vi "Read.vi"(6 "prioritize Cache? (F)":bool, 7 "Qualified Name":string, 8 "error in (no error)":errorcluster, 9 "Default Values":variant[](array[variant]), 10 "keys in":string[](array[string]), 11 "ConfigManager in":refnum<class "ConfigManager.lvclass">) -> (0 "error out":errorcluster, 1 "Values":variant[](array[variant]), 2 "keys":string[](array[string]), 3 "ConfigManager out":refnum<class "ConfigManager.lvclass">)   [LabVIEW 2013, in "CfgManager.lvlib" / "ConfigManager.lvclass"]
uses:
  ConfigManager.lvclass
  ConfigManager.lvclass/ConfigManager.ctl
  Encoding/Encoding.lvclass
  Encryption/Encryption.lvclass
  Serializer/Serializer.lvclass
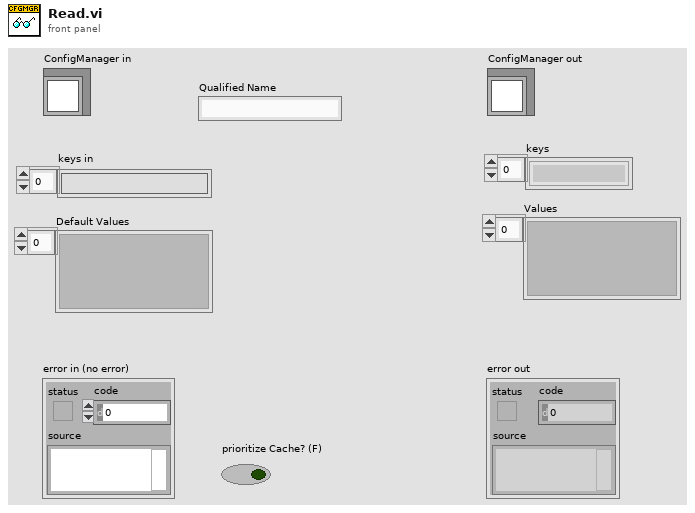
[diagram p1: front panel]
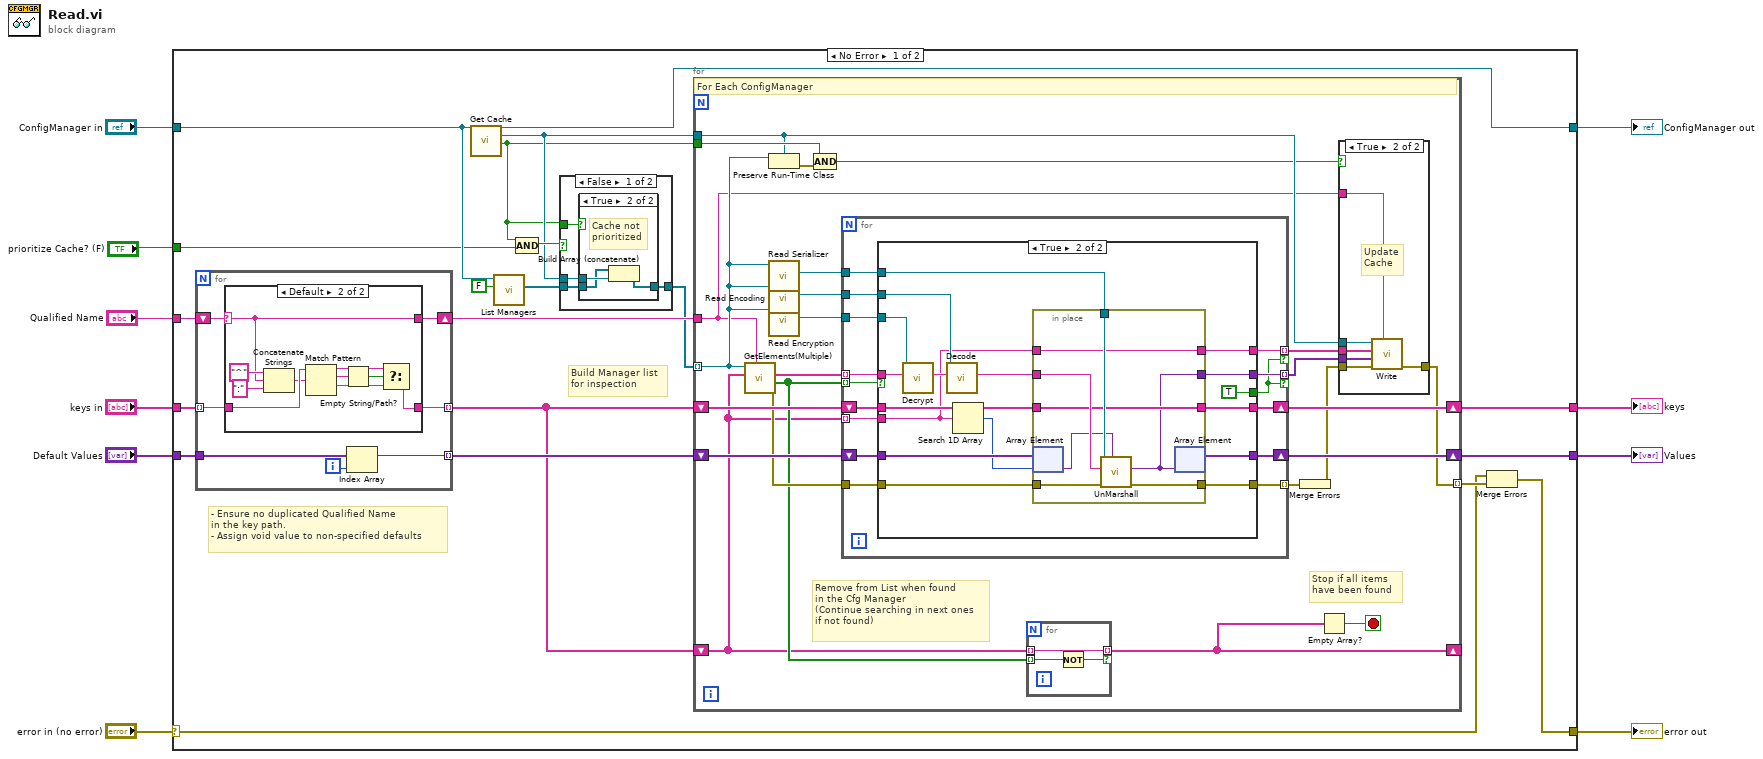
[diagram p0: block diagram]
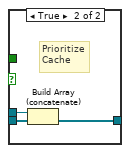
[diagram p3: hidden frame]
diagram:
  n1 = case shown="No Error" "error in (no error)" {
    selector: "error in (no error)" -> [w25 w141]
    tunnel: [w24 w141] -> w9
    tunnel: [w11 w140] -> w7
    tunnel: "ConfigManager in" -> [w18 w140]
    tunnel: "keys in" -> [w23 w138]
    tunnel: "Default Values" -> [w29 w139]
    tunnel: [w28 w139] -> w4
    tunnel: [w27 w138] -> w3
    tunnel: "Qualified Name" -> [w21 _]
    tunnel: "prioritize Cache? (F)" -> [w14 _]
    frame No Error {
      # "Build Manager list\nfor inspection"
      # "- Ensure no duplicated Qualified Name\nin the key path.\n- Assign void value to non-specified defaults"
      n2 = for {
        tunnel: w29 -> [w47]
        tunnel: [w46] -> w30 mode=indexing
        tunnel: w23 -> [w45] mode=indexing
        tunnel: [w42] -> w22 mode=indexing
        shift-right: [w43] -> w20
        shift-left: w21 -> [w44]
        i -> [w48]
        n3 = case shown="Default" w44 {
          selector: w44 -> [w50 w57]
          tunnel: w45 -> [w49 w60]
          tunnel: [w50 w57] -> w43
          tunnel: [w49 w51] -> w42
          frame "" {
          }
          frame Default {
            n4 = Concatenate Strings("^" ("string"), w57, ":" ("string")) -> (w59:string)
            n5 = Match Pattern(string=w60, regular expression=w59) -> (before substring=w54:string, match substring=w56:string, after substring=w53:string)  [unwired: 1 in, 1 out]
            n6 = Empty String/Path?(string/path=w56) -> (empty?=w55:bool)
            n7 = Select(t=w54, s=w55, f=w53) -> (s? t:f=w51:string)
          }
        }
        n8 = Index Array(array=w47, index=w48) -> (element=w46:variant)
      }
      n9 = call-dynamic "Get Cache.vi"("ConfigManager in"=w18) -> ("found?"=w12:bool, "Cache"=w13:refnum<class "ConfigManager.Cache.lvclass">, "ConfigManager out"=w11:refnum<class "ConfigManager.lvclass">)  [unwired: 8 in]
      n10 = call-dynamic "List Managers.vi"("Include Cache? (F)"=FALSE, "ConfigManager in"=w18) -> ("List"=w17:refnum<class "ConfigManager.lvclass">[])  [unwired: 8 in, 1 out]
      n11 = Compound Arithmetic op=AND(w12, w14) -> (w15:bool)
      n12 = case shown="False" w15 {
        tunnel: w13 -> [w33 w41]
        tunnel: w17 -> [w32 w40]
        tunnel: [w31 w39] -> w16
        tunnel: w12 -> [w34 _]
        frame False {
          n13 = case shown="True" w34 {
            tunnel: w33 -> [_ w38]
            tunnel: w32 -> [w35 w37]
            tunnel: [w35 w36] -> w31
            frame False {
              # "No cache\nfound"
            }
            frame True {
              # "Cache not\nprioritized"
              n14 = Build Array (concatenate)(w37, w38) -> (w36:refnum<class "ConfigManager.lvclass">[])
            }
          }
        }
        frame True {
          # "Prioritize\nCache"
          n15 = Build Array (concatenate)(w41, w40) -> (w39:refnum<class "ConfigManager.lvclass">[])
        }
      }
      n16 = for {
        tunnel: w16 -> [w75] mode=indexing
        shift-right: [w61] -> _
        shift-left: w22 -> [w63]
        shift-right: [w80] -> w28
        shift-left: w30 -> [w83]
        shift-right: [w81] -> w27
        shift-left: w22 -> [w82]
        tunnel: [w69] -> w26 mode=indexing
        tunnel: w20 -> [w67]
        tunnel: w13 -> [w72]
        tunnel: w12 -> [w73]
        stop <- w62 stop-if-true
        # "Remove from List when found\nin the Cfg Manager\n(Continue searching in next ones\nif not found)"
        # "Stop if all items\nhave been found"
        # "For Each ConfigManager"
        n17 = call-dynamic "GetElements(Multiple).vi"("Qualified Name"=w67, "keys"=w63, "ConfigManager in"=w75) -> ("error out"=w65:errorcluster, "Found"=w64:bool[], "Values"=w84:string[])  [unwired: 5 in, 1 out]
        n18 = Preserve Run-Time Class(object in=w75, 2:w72) -> (error out=w74:errorcluster)  [unwired: 1 in, 1 out]
        n19 = call "Read Serializer.vi"("ConfigManager in"=w75) -> ("Serializer"=w78:refnum<class "Serializer.lvclass">)  [unwired: 9 in, 1 out]
        n20 = call "Read Encoding.vi"("ConfigManager in"=w75) -> ("Encoding"=w79:refnum<class "Encoding.lvclass">)  [unwired: 9 in, 1 out]
        n21 = call "Read Encryption.vi"("ConfigManager in"=w75) -> ("Encryption"=w76:refnum<class "Encryption.lvclass">)  [unwired: 9 in, 1 out]
        n22 = Compound Arithmetic op=AND(w73, w74) -> (w66:bool)
        n23 = for {
          tunnel: w84 -> [w109] mode=indexing
          tunnel: w78 -> [w108]
          tunnel: w79 -> [w107]
          tunnel: w64 -> [w106] mode=indexing
          shift-right: [w103] -> w81
          shift-left: w82 -> [w105]
          shift-right: [w102] -> w80
          shift-left: w83 -> [w104]
          tunnel: w65 -> [w101]
          tunnel: [w100] -> w77 mode=indexing
          tunnel: w63 -> [w99] mode=indexing
          tunnel: w76 -> [w98]
          tunnel: [w97] -> w70 mode=indexing if=w95
          tunnel: [w96] -> w71 mode=indexing if=w95
          n24 = case shown="True" w106 {
            tunnel: w109 -> [_ w119]
            tunnel: w108 -> [_ w125]
            tunnel: w107 -> [_ w129]
            tunnel: w105 -> [w112 w122]
            tunnel: w104 -> [w111 w128]
            tunnel: [w112 w123] -> w103
            tunnel: [w111 w127] -> w102
            tunnel: w101 -> [w110 w121]
            tunnel: [w110 w120] -> w100
            tunnel: w99 -> [_ w114]
            tunnel: w98 -> [_ w117]
            tunnel: [_ w116] -> w97
            tunnel: [_ w115] -> w96
            tunnel: [_ TRUE] -> w95
            frame False {
            }
            frame True {
              n25 = call-dynamic "Decrypt.vi"("Encrypted String"=w119, "Encryption in"=w117) -> ("String"=w118:string)  [unwired: 8 in, 1 out]
              n26 = call-dynamic "Decode.vi"("Encoded String"=w118, "CfgEncoding in"=w129) -> ("String"=w124:string)  [unwired: 8 in, 1 out]
              n27 = Search 1D Array(1D array=w122, element=w114) -> (index of element=w126:i32)  [unwired: 1 in]
              n28 = in-place {
                in-place-border: w125 -> [w137]
                in-place-border: w124 -> [w136]
                in-place-border: [w134] -> w123
                in-place-border: w122 -> [w134]
                in-place-border: w121 -> [w133]
                in-place-border: [w132] -> w120
                in-place-border: [w131] -> w116
                in-place-border: [w130] -> w115
                in-place-border: w114 -> [w130]
                n29 = in-place-array #1(w128, w126) -> (w135:variant)
                n30 = call-dynamic "UnMarshall.vi"("Type"=w135, "error in (no error)"=w133, "String"=w136, "Serializer in"=w137) -> ("error out"=w132:errorcluster, "Variant"=w131:variant)  [unwired: 5 in, 1 out]
                n31 = in-place-array #1(w131) -> (w127:variant[])  [unwired: 1 out]
              }
            }
          }
        }
        n32 = for {
          tunnel: w63 -> [w94] mode=indexing
          tunnel: w64 -> [w93] mode=indexing
          tunnel: [w94] -> w61 mode=indexing if=w92
          n33 = Not(x=w93) -> (.not. x?=w92:bool)
        }
        n34 = Merge Errors(w77) -> (w68:errorcluster)
        n35 = Empty Array?(array=w61) -> (empty?=w62:bool)
        n36 = case shown="True" w66 {
          tunnel: w72 -> [_ w91]
          tunnel: w71 -> [_ w90]
          tunnel: w70 -> [_ w89]
          tunnel: [w85 w86] -> w69
          tunnel: w68 -> [w85 w88]
          tunnel: w67 -> [_ w87]
          frame False {
          }
          frame True {
            # "Update\nCache"
            n37 = call "Write.vi"("Qualified Name"=w87, "error in (no error)"=w88, "Values"=w89, "keys"=w90, "ConfigManager in"=w91) -> ("error out"=w86:errorcluster)  [unwired: 4 in, 2 out]
          }
        }
      }
      n38 = Merge Errors(w25, w26) -> (w24:errorcluster)
    }
    frame Error {
    }
  }
  "error out" <- w9
  "ConfigManager out" <- w7
  "Values" <- w4
  "keys" <- w3
